vi "svc_Check Frequency Range in Bandwidth.vi"(8 "fmax":dbl, 9 "fmin":dbl, 11 "frequency range":T1) -> (0 "start and stop in range":bool, 1 "zero span":bool, 2 "stop frequency":dbl, 3 "start frequency":dbl)   [LabVIEW 2017]
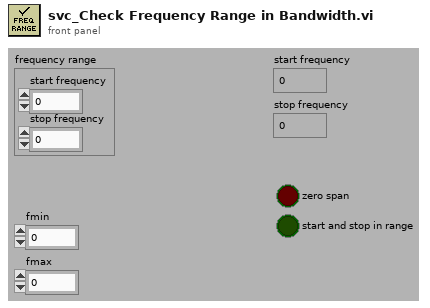
[diagram p1: front panel]
types:
  T1 = cluster{"start frequency":dbl, "stop frequency":dbl}
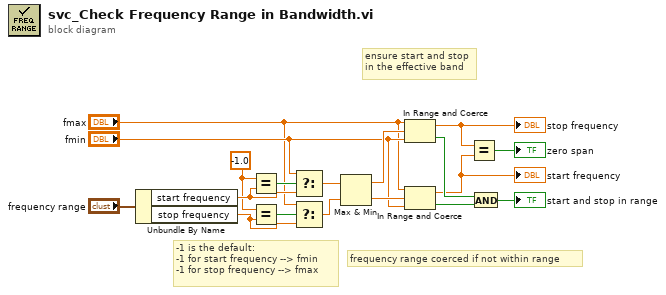
[diagram p0: block diagram]
diagram:
  w16 = -1.0 ("x")
  # "frequency range coerced if not within range"
  # "ensure start and stop\nin the effective band"
  # "-1 is the default:\n-1 for start frequency --> fmin\n-1 for stop frequency --> fmax"
  n1 = Unbundle By Name("frequency range") -> ("start frequency"=w17:dbl, "stop frequency"=w18:dbl)
  n2 = Equal?(x=w16, y=w17) -> (x = y?=w14:bool)
  n3 = Equal?(x=w16, y=w18) -> (x = y?=w15:bool)
  n4 = Select(t="fmin", s=w14, f=w17) -> (s? t:f=w8:dbl)
  n5 = Select(t="fmax", s=w15, f=w18) -> (s? t:f=w7:dbl)
  n6 = Max & Min(x=w8, y=w7) -> (max(x,y)=w6:dbl, min(x,y)=w5:dbl)
  n7 = In Range and Coerce(upper limit="fmax", x=w6, lower limit="fmin") -> (coerced(x)=w3:dbl, In Range?=w9:bool)
  "stop frequency" <- w3
  n8 = In Range and Coerce(upper limit="fmax", x=w5, lower limit="fmin") -> (coerced(x)=w4:dbl, In Range?=w10:bool)
  "start frequency" <- w4
  n9 = Equal?(x=w3, y=w4) -> (x = y?=→"zero span":bool)
  n10 = And(x=w9, y=w10) -> (x .and. y?=→"start and stop in range":bool)
